vi "Next.vi"(8 "error in (no error)":errorcluster, 11 "Iterate in":refnum<class "Abs_Waveform.lvclass">) -> (0 "error out":errorcluster, 2 "Last?":bool, 3 "Iterate out":refnum<class "Abs_Waveform.lvclass">)   [LabVIEW 2021, in "Abs_Waveform.lvclass"]
uses:
  Abs_Waveform.lvclass
  Abs_Waveform.lvclass/Abs_Waveform.ctl
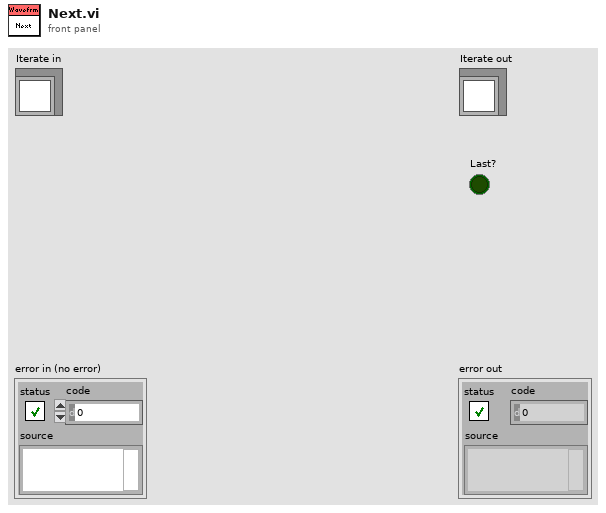
[diagram p1: front panel]
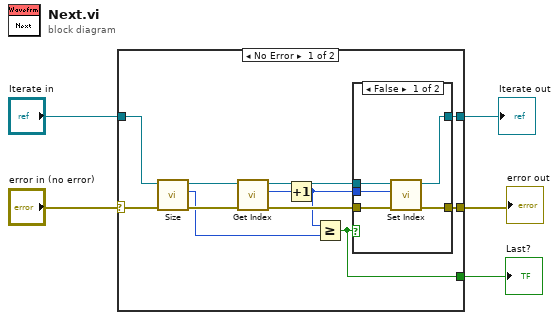
[diagram p0: block diagram]
diagram:
  n1 = case shown="No Error" "error in (no error)" {
    selector: "error in (no error)" -> [w9 w25]
    tunnel: [w16 w26] -> w5
    tunnel: "Iterate in" -> [w12 w26]
    tunnel: [w10 w25] -> w3
    tunnel: [w6 _] -> w1
    frame No Error {
      n2 = call-dynamic "Size.vi"("error in (no error)"=w9, "Abs_Waveform in"=w12) -> ("error out"=w11:errorcluster, "size"=w7:i32, "Abs_Waveform out"=w13:refnum<class "Abs_Waveform.lvclass">)  [unwired: 7 in]
      n3 = call-dynamic "Get Index.vi"("error in (no error)"=w11, "Abs_Waveform in"=w13) -> ("error out"=w15:errorcluster, "Index"=w14:i32, "Abs_Waveform out"=w17:refnum<class "Abs_Waveform.lvclass">)  [unwired: 7 in]
      n4 = Increment(x=w14) -> (x+1=w8:i32)
      n5 = Greater Or Equal?(x=w8, y=w7) -> (x >= y?=w6:bool)
      n6 = case shown="False" w6 {
        tunnel: w17 -> [w22 w24]
        tunnel: [w21 w24] -> w16
        tunnel: w15 -> [w20 w23]
        tunnel: w8 -> [w19 _]
        tunnel: [w18 w23] -> w10
        frame False {
          n7 = call-dynamic "Set Index.vi"("error in (no error)"=w20, "Index"=w19, "Abs_Waveform in"=w22) -> ("error out"=w18:errorcluster, "Abs_Waveform out"=w21:refnum<class "Abs_Waveform.lvclass">)  [unwired: 7 in]
        }
        frame True {
        }
      }
    }
    frame Error {
    }
  }
  "error out" <- w3
  "Iterate out" <- w5
  "Last?" <- w1
